vi "comm timeout2.vi"(5 "ulReadIntervalTimeout":u32, 6 "ulWriteTotalTimeoutMultiplier":u32, 7 "ulReadTotalTimeoutMultiplier":u32, 8 "error in (no error)":errorcluster, 9 "ulWriteTotalTimeoutConstant":u32, 10 "ulReadTotalTimeoutConstant":u32, 11 "Comm Handle":u32) -> (0 "error out":errorcluster, 3 "dup Comm Handle":u32)   [LabVIEW 2013, in "lvserial.lvlib"]
doc: "Configures the timeout value for read and write operations."
uses:
  lvserial.lvlib
  lvserial.dll
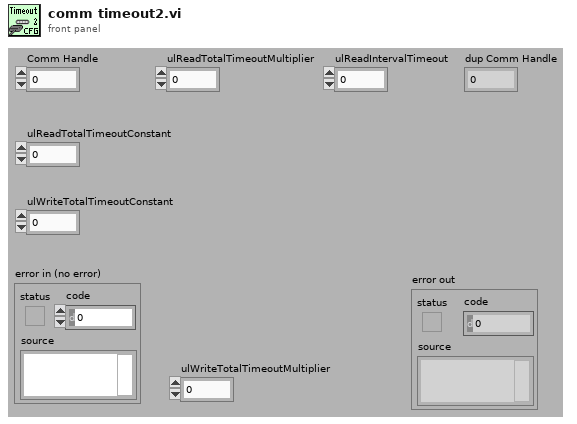
[diagram p1: front panel]
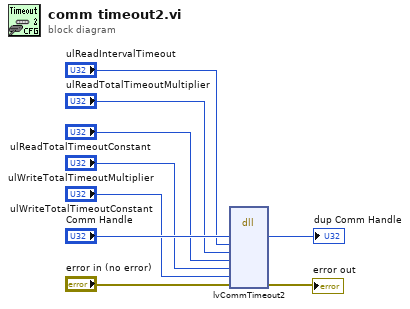
[diagram p0: block diagram]
diagram:
  n1 = dll-call lib="lvserial.dll" fn="lvCommTimeout2"("hComm"="Comm Handle", "ulReadIntervalTimeout"="ulReadIntervalTimeout", "ulReadTotalTimeoutMultiplier"="ulReadTotalTimeoutMultiplier", "ulReadTotalTimeoutConstant"="ulReadTotalTimeoutConstant", "ulWriteTotalTimeoutMultiplier"="ulWriteTotalTimeoutMultiplier", "ulWriteTotalTimeoutConstant"="ulWriteTotalTimeoutConstant", "error in (no error)"="error in (no error)") -> ("hComm"=→"dup Comm Handle":u32, "error in (no error)"=→"error out":errorcluster)  [unwired: 8 in, 3 out]
